vi "Time to End.vi"(6 "Trigger":variant, 7 "Start Time (ms)":u32, 8 "i":i32, 11 "N":i32) -> (0 "Time To End (min)":dbl, 1 "Time To End (s)":dbl, 2 "Time to End":cluster{"Time To End":dbl, "unit":string} {"Time To End" format="%#_4g"}, 3 "Percent Complete":dbl(slide) scale=0.0..1.0, 4 "Time To End (hr)":dbl)   [LabVIEW 2019]
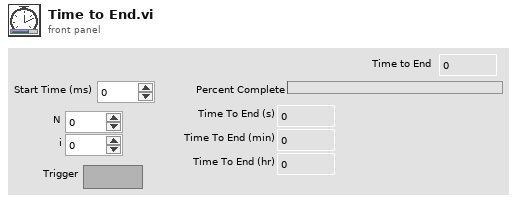
[diagram p1: front panel]
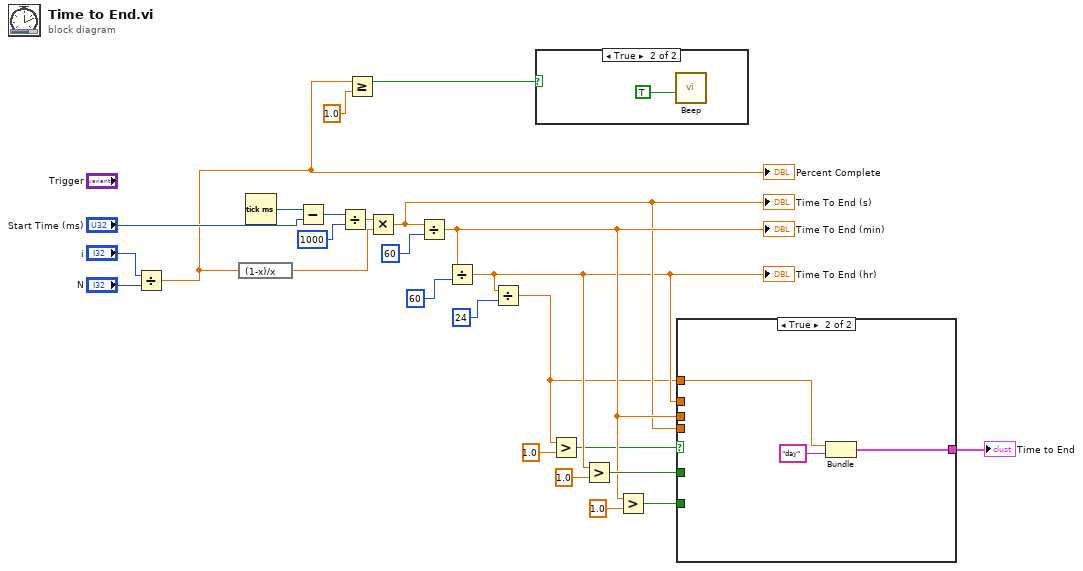
[diagram p0: block diagram]
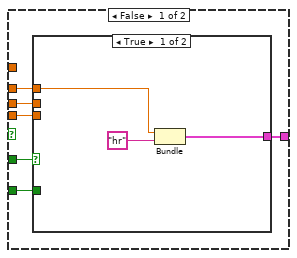
[diagram p2: hidden frame]
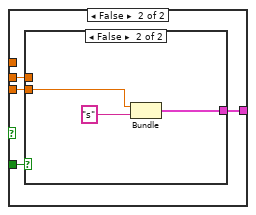
[diagram p3: hidden frame]
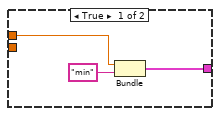
[diagram p4: hidden frame]
diagram:
  n1 = Divide(x="i", y="N") -> (x/y=w15:dbl)
  "Percent Complete" <- w15
  n2 = expression code="(1-x)/x"(w15) -> (w22:dbl)
  n3 = Tick Count (ms)() -> (millisecond timer value=w24:u32)
  n4 = Subtract(x=w24, y="Start Time (ms)") -> (x-y=w19:u32)
  n5 = Divide(x=w19, y=u32 1000) -> (x/y=w20:dbl)
  n6 = Greater Or Equal?(x=w15, y=1.0) -> (x >= y?=w7:bool)
  n7 = Multiply(x=w20, y=w22) -> (x*y=w8:dbl)
  "Time To End (s)" <- w8
  n8 = Divide(x=w8, y=u32 60) -> (x/y=w9:dbl)
  "Time To End (min)" <- w9
  n9 = Divide(x=w9, y=u32 60) -> (x/y=w5:dbl)
  "Time To End (hr)" <- w5
  n10 = Divide(x=w5, y=u32 24) -> (x/y=w1:dbl)
  n11 = case shown="True" w7 {
    frame False {
    }
    frame True {
      n12 = call <vilib>:"Beep.vi"("use system alert? (T)"=TRUE) -> ()  [unwired: 11 in]
    }
  }
  n13 = Greater?(x=w1, y=1.0) -> (0:w2:bool)
  n14 = Greater?(x=w5, y=1.0) -> (0:w13:bool)
  n15 = Greater?(x=w9, y=1.0) -> (0:w10:bool)
  n16 = case shown="True" w2 {
    tunnel: w13 -> [w32 _]
    tunnel: w5 -> [w31 _]
    tunnel: [w30 w47] -> w12
    tunnel: w10 -> [w29 _]
    tunnel: w9 -> [w28 _]
    tunnel: w8 -> [w27 _]
    tunnel: w1 -> [_ w46]
    frame False {
      n17 = case shown="True" w32 {
        tunnel: w31 -> [w35 _]
        tunnel: [w33 w39] -> w30
        tunnel: w29 -> [_ w38]
        tunnel: w28 -> [_ w37]
        tunnel: w27 -> [_ w36]
        frame True {
          n18 = Bundle(w35, "hr") -> (w33:cluster{dbl, string})  [unwired: 1 in]
        }
        frame False {
          n19 = case shown="False" w38 {
            tunnel: w37 -> [w42 _]
            tunnel: [w40 w44] -> w39
            tunnel: w36 -> [_ w43]
            frame True {
              n20 = Bundle(w42, "min") -> (w40:cluster{dbl, string})  [unwired: 1 in]
            }
            frame False {
              n21 = Bundle(w43, "s") -> (w44:cluster{dbl, string})  [unwired: 1 in]
            }
          }
        }
      }
    }
    frame True {
      n22 = Bundle(w46, "day") -> (w47:cluster{dbl, string})  [unwired: 1 in]
    }
  }
  "Time to End" <- w12
